vi "Startup.vi"(6 "LabVIEW Web Service":refnum<class "Web Service.lvclass">) -> ()   [LabVIEW 2017]
uses:
  <vilib>/wsapi/Web Service.lvclass
  <vilib>/Utility/config.llb/Read Key (Boolean).vi
  <vilib>/Utility/config.llb/Read Key (I32).vi
  <vilib>/Utility/tcp.llb/UDP Multicast Read-Only Open.vi
  <vilib>/Utility/config.llb/NI_LVConfig.lvlib
panel:
  in  "stop":bool
  out "error out":errorcluster
  # "Use the web service input terminal to call the VIs on the Service subpalette of the Web Services palette. Do not remove it from the connector pane unless you don't need access to the palette."
  # "Any additional terminals added to the connector pane of a startup VI will be ignored."
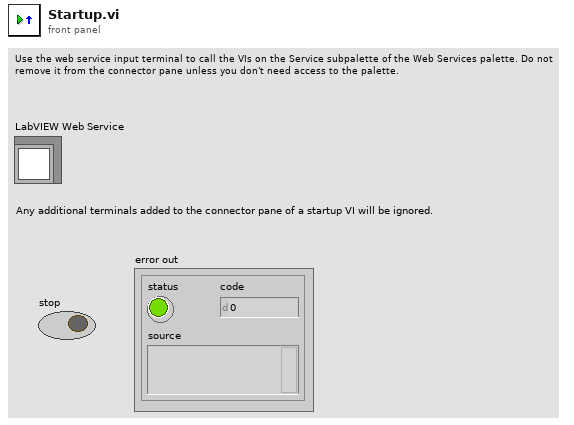
[diagram p1: front panel]
types:
  T1 = typedef "NI_LVConfig.lvlib/Config Data RefNum.ctl" = refnum<k1>
  T2 = typedef "cmdSetup.ctl" = cluster{"DefaultQueueName":string, "responseTimeout":i32, "logPostdata":string, "logResponse":string}
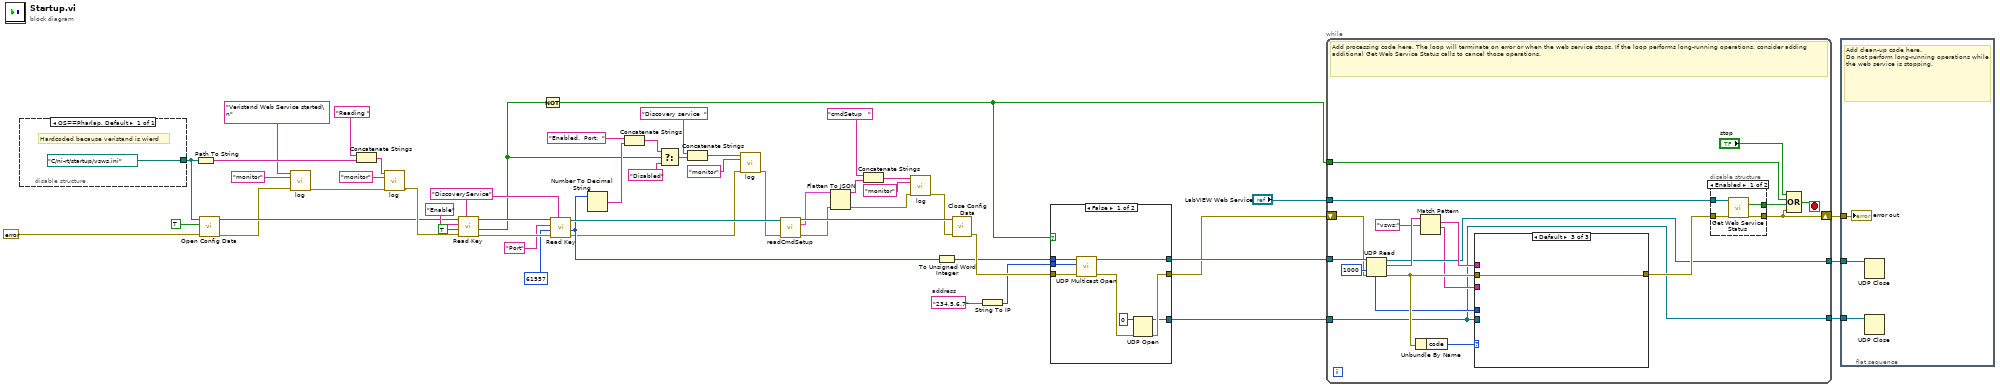
[diagram p0: block diagram]
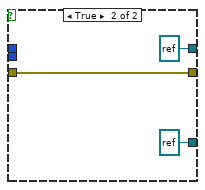
[diagram p2: hidden frame]
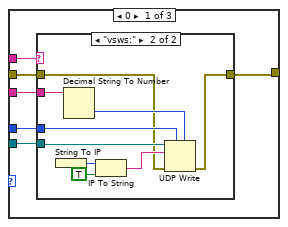
[diagram p4: hidden frame]
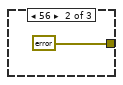
[diagram p6: hidden frame]
diagram:
  w22 = "234.5.6.7"  # address
  w35 = "DiscoveryService" ("section")
  n1 = disable-structure shown="OS==Pharlap, Default" {
    disable-tunnel: [path "C:/ni-rt/startup/vsws.ini" ("configuration file path")] -> w1
    frame condition #0 (active) {
      # "Hardcoded because veristand is wierd"
    }
  }
  n2 = Path To String(path=w1) -> (string=w48:string)
  n3 = call <vilib>:"Open Config Data.vi"("error in (no error)"=errorcluster {"status"=FALSE, "code"=0, "source"=""} ("error constant"), "create file if necessary (T)"=TRUE, "configuration file path"=w1) -> ("error out"=w11:errorcluster, "refnum"=w12:T1)  [unwired: 6 in, 1 out]
  n4 = call "log.vi"("log string"="Veristand Web Service started\n" ("String to write"), "logOption"="monitor", "error in (no error)"=w11) -> ("error out"=w16:errorcluster)  [unwired: 12 in]
  n5 = Concatenate Strings("Reading " ("string"), w48) -> (w15:string)
  n6 = call "log.vi"("log string"=w15, "logOption"="monitor", "error in (no error)"=w16) -> ("error out"=w13:errorcluster)  [unwired: 12 in]
  n7 = call-poly <vilib>:"Read Key.vi"("section"=w35, "error in (no error)"=w13, "default value"=TRUE, "key"="Enable", "refnum"=w12) -> ("error out"=w37:errorcluster, "value"=w27:bool, "refnum out"=w38:T1)  [unwired: 3 in, 1 out]
  n8 = Not(x=w27) -> (.not. x?=w23:bool)
  n9 = call-poly <vilib>:"Read Key.vi"("section"=w35, "error in (no error)"=w37, "default value"=61557, "key"="Port", "refnum"=w38) -> ("error out"=w9:errorcluster, "value"=w25:i32, "refnum out"=w36:T1)  [unwired: 3 in, 1 out]
  n10 = Number To Decimal String(number=w25) -> (decimal integer string=w31:string)  [unwired: 1 in]
  n11 = Concatenate Strings("Enabled.  Port:  " ("string"), w31) -> (w28:string)
  n12 = Select(t=w28, s=w27, f="Disabled") -> (s? t:f=w46:string)
  n13 = Concatenate Strings("Discovery service  " ("string"), w46) -> (w10:string)
  n14 = call "log.vi"("log string"=w10, "logOption"="monitor", "error in (no error)"=w9) -> ("error out"=w8:errorcluster)  [unwired: 12 in]
  n15 = call "readCmdSetup.vi"("refnum in"=w36, "error in (no error)"=w8) -> ("refnum out"=w43:T1, "cmdSetup"=w42:T2, "error out"=w41:errorcluster)  [unwired: 11 in]
  n16 = Flatten To JSON(anything=w42, error in (no error)=w41) -> (JSON string=w6:string, 11:w4:errorcluster)  [unwired: 1 in]
  n17 = Concatenate Strings("cmdSetup   " ("string"), w6) -> (w5:string)
  n18 = call "log.vi"("log string"=w5, "logOption"="monitor", "error in (no error)"=w4) -> ("error out"=w3:errorcluster)  [unwired: 12 in]
  n19 = To Unsigned Word Integer(number=w25) -> (unsigned 16bit integer=w24:u16)
  n20 = call <vilib>:"Close Config Data.vi"("error in (no error)"=w3, "refnum"=w43) -> ("error out"=w39:errorcluster)  [unwired: 8 in, 1 out]
  n21 = String To IP(1:w22) -> (0:w21:u32)
  n22 = case shown="False" w23 {
    tunnel: w39 -> [w63 w66]
    tunnel: [w62 refnum<k16> refnum ("port")] -> w30
    tunnel: [w57 w66] -> w29
    tunnel: w24 -> [w61 _]
    tunnel: w21 -> [w60 _]
    tunnel: [w56 refnum<k16> refnum ("port")] -> w20
    frame False {
      n23 = call-poly <vilib>:"UDP Multicast Open.vi"("error in (no error)"=w63, "multicast addr"=w60, "port"=w61) -> ("error out"=w58:errorcluster, "connection ID"=w62:refnum<k16>)  [unwired: 6 in, 1 out]
      n24 = UDP Open(8:w58, 11:u16 0 ("port")) -> (port=w56:refnum<k16>, 0:w57:errorcluster)  [unwired: 3 in, 1 out]
    }
    frame True {
    }
  }
  n25 = while {
    tunnel: "LabVIEW Web Service" -> [w83]
    shift-right: [w84] -> w52
    shift-left: w29 -> [w78]
    tunnel: w30 -> [w82]
    tunnel: [w69] -> w26
    tunnel: w23 -> [w74]
    tunnel: w20 -> [w67]
    tunnel: [w67] -> w19
    stop <- w85 stop-if-true
    # "Add processing code here. The loop will terminate on error or when the web service stops. If the loop performs long-running operations, consider adding additional Get Web Service Status calls to cancel those operations."
    n26 = UDP Read(connection ID=w82, timeout ms (25000)=1000, 8:w78) -> (data out=w72:string, error out=w79:errorcluster, 3:w69:refnum<k16>, 6:w75:u32)  [unwired: 1 in, 1 out]
    n27 = Unbundle By Name(w79) -> ("code"=w81:i32)
    n28 = Match Pattern(string=w72, regular expression="vsws:") -> (match substring=w70:string, after substring=w68:string)  [unwired: 1 in, 2 out]
    n29 = case shown="Default" w81 {
      tunnel: w70 -> [w96 _ _]
      tunnel: w79 -> [w95 _ w108]
      tunnel: [w94 errorcluster {"status"=FALSE, "code"=0, "source"=""} ("error out") w108] -> w77
      tunnel: w75 -> [w93 _ _]
      tunnel: w67 -> [w92 _ _]
      tunnel: w68 -> [w91 _ _]
      frame 0 {
        n30 = case shown="\"vsws:\"" w96 {
          tunnel: w95 -> [w97 w99]
          tunnel: [w97 w98] -> w94
          tunnel: w93 -> [_ w102]
          tunnel: w92 -> [_ w103]
          tunnel: w91 -> [_ w101]
          frame Default {
          }
          frame "vsws:" {
            n31 = String To IP() -> (0:w106:u32)  [unwired: 1 in]
            n32 = Decimal String To Number(string=w101) -> (number=w100:i32)  [unwired: 2 in, 1 out]
            n33 = IP To String(1:TRUE ("dot notation? (F)"), 2:w106) -> (0:w104:string)
            n34 = UDP Write(address=w102, port or service name=w100, connection ID=w103, data in=w104, 8:w99) -> (error out=w98:errorcluster)  [unwired: 1 in, 1 out]
          }
        }
      }
      frame 56 {
      }
      frame Default {
      }
    }
    n35 = disable-structure shown="Enabled" {
      disable-tunnel: [w89 w90] -> w84
      disable-tunnel: w83 -> [w88 _]
      disable-tunnel: w77 -> [w87 w90]
      disable-tunnel: [w86 _] -> w76
      frame Enabled {
        n36 = call <vilib>:"Get Web Service Status.vi"("LabVIEW Web Service"=w88, "error in (no error)"=w87) -> ("service stopping?"=w86:bool, "error out"=w89:errorcluster)  [unwired: 11 in, 1 out]
      }
      frame Disabled {
      }
    }
    n37 = Compound Arithmetic op=OR("stop", w74, w76, w84) -> (w85:bool)
  }
  n38 = flat-sequence {
    tunnel: w52 -> [w110]
    tunnel: w26 -> [w111]
    tunnel: w19 -> [w109]
    frame #0 {
      # "Add clean-up code here.\nDo not perform long-running operations while the web service is stopping."
      n39 = UDP Close(connection ID=w111) -> ()  [unwired: 1 in, 2 out]
      n40 = UDP Close(connection ID=w109) -> ()  [unwired: 1 in, 2 out]
      "error out" <- w110
    }
  }
